vi "Pockels-Convert AO sequence from time to samples.vi"(8 "Direction (+Inf)":T1=enum."Toward +Inf", 11 "Duration of AO sequence (us)":dbl format="%#_6f") -> (3 "Number of samples in AO sequence":i32)   [LabVIEW 2020]
uses:
  Typedefs/Rounding type.ctl
  Global Variables/General Globals.vi
panel:
  out "Sampling period (us)":dbl
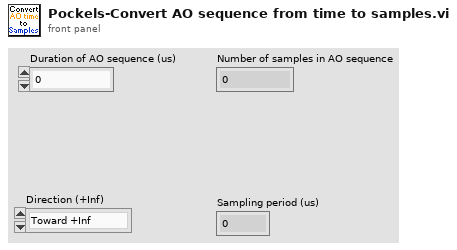
[diagram p1: front panel]
types:
  T1 = typedef "Rounding type.ctl" = enum16{"No rounding", "Toward +Inf", "Toward -Inf"}
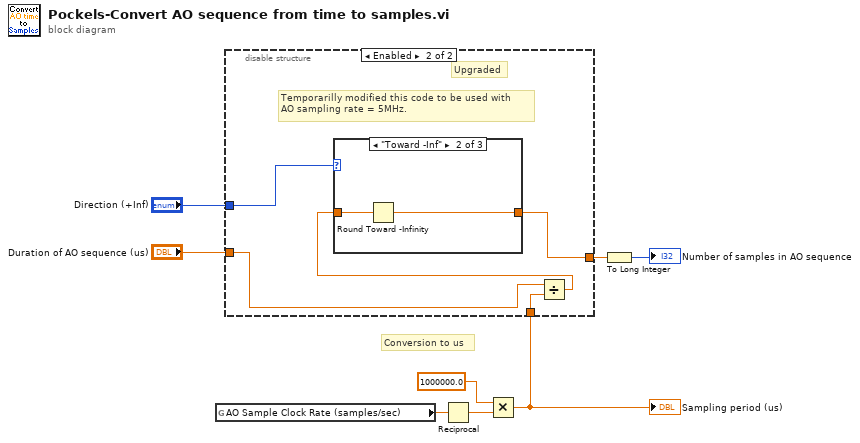
[diagram p0: block diagram]
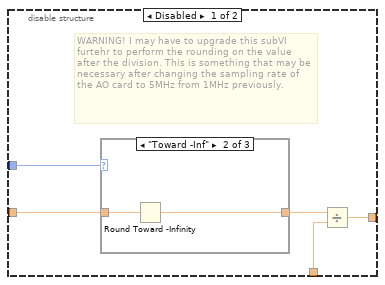
[diagram p2: hidden frame]
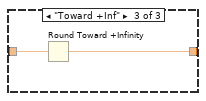
[diagram p4: hidden frame]
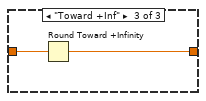
[diagram p6: hidden frame]
diagram:
  # "Conversion to us"
  n1 = global read "General Globals.vi" "AO Sample Clock Rate (samples/sec)"() -> (w1:dbl)
  n2 = Reciprocal(x=w1) -> (1/x=w7:dbl)
  n3 = Multiply(x=1000000.0 ("y"), y=w7) -> (x*y=w6:dbl)
  "Sampling period (us)" <- w6
  n4 = disable-structure shown="Enabled" {
    disable-tunnel: [w13 w19] -> w8
    disable-tunnel: w6 -> [w12 w23]
    disable-tunnel: "Duration of AO sequence (us)" -> [w11 w21]
    disable-tunnel: "Direction (+Inf)" -> [w9 w22]
    frame Disabled {
      # "WARNING! I may have to upgrade this subVI furtehr to perform the rounding on the value after the division. This is something that may be necessary after changing the sampling rate of the AO card to 5MHz from 1MHz previously."
      n5 = case shown="\"Toward -Inf\"" w9 {
        tunnel: w11 -> [w14 w16 w18]
        tunnel: [w14 w15 w17] -> w10
        frame "No rounding", Default {
        }
        frame "Toward -Inf" {
          n6 = Round Toward -Infinity(1:w16) -> (0:w15:dbl)
        }
        frame "Toward +Inf" {
          n7 = Round Toward +Infinity(x=w18) -> (ceil(x): smallest int >= x=w17:dbl)
        }
      }
      n8 = Divide(x=w10, y=w12) -> (x/y=w13:dbl)
    }
    frame Enabled {
      # "Upgraded"
      # "Temporarilly modified this code to be used with\nAO sampling rate = 5MHz."
      n9 = Divide(x=w21, y=w23) -> (x/y=w20:dbl)
      n10 = case shown="\"Toward -Inf\"" w22 {
        tunnel: w20 -> [w24 w26 w28]
        tunnel: [w24 w25 w27] -> w19
        frame "No rounding", Default {
        }
        frame "Toward -Inf" {
          n11 = Round Toward -Infinity(1:w26) -> (0:w25:dbl)
        }
        frame "Toward +Inf" {
          n12 = Round Toward +Infinity(x=w28) -> (ceil(x): smallest int >= x=w27:dbl)
        }
      }
    }
  }
  n13 = To Long Integer(number=w8) -> (32bit integer=→"Number of samples in AO sequence":i32)
